vi "GoToWavelength.vi"(8 "error in (no error)":errorcluster, 10 "Wavelength":dbl, 11 "HRS_Spectrometer in":refnum<class "HRS_Spectrometer.lvclass">) -> (0 "error out":errorcluster, 3 "HRS_Spectrometer out":refnum<class "HRS_Spectrometer.lvclass">)   [LabVIEW 2023, in "HRS_Spectrometer.lvlib" / "HRS_Spectrometer.lvclass"]
uses:
  HRS_Spectrometer.lvclass
  HRS_Spectrometer.lvclass/HRS_Spectrometer.ctl
  <vilib>/Instr/_visa.llb/Select Event Type.ctl
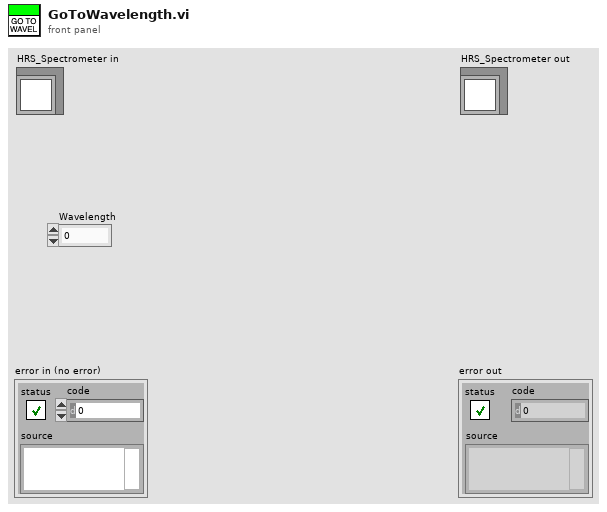
[diagram p1: front panel]
types:
  T1 = typedef "Select Event Type.ctl" = u32
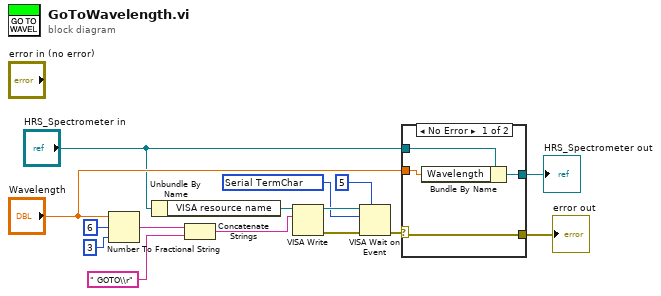
[diagram p0: block diagram]
diagram:
  w4 = T1 1073684516 items=["Service Request"=1073684491, "Trigger"=3221168138, "Clear"=1073684493, "VXI Signal"=1073684512, "VXI/VME Interrupt"=3221168161, "VXI/VME Sysfail"=1073684509, "VXI/VME Sysreset"=1073684510, "GPIB CIC"=1073684498, "GPIB Talk"=1073684499, "GPIB Listen"=1073684500, "PXI Interrupt"=1073684514, "Serial Break"=1073684515, "Serial TermChar"=1073684516, "Serial CTS"=1073684521, "Serial DSR"=1073684522, "Serial DCD"=1073684524, "Serial RI"=1073684526, "Serial Character"=1073684533, "USB Interrupt"=1073684535, "All Enabled"=1073709055] ("Event Type")
  n1 = Number To Fractional String(number="Wavelength", width (-)=i16 6, precision (6)=i16 3) -> (F-format string=w8:string)  [unwired: 1 in]
  n2 = Unbundle By Name("HRS_Spectrometer in") -> ("VISA resource name"=w10:refnum<visa-resource-name>)
  n3 = Concatenate Strings(w8, " GOTO\\r") -> (w7:string)
  n4 = VISA Write(VISA resource name=w10, write buffer=w7) -> (VISA resource name out=w6:refnum<visa-resource-name>, error out=w3:errorcluster)  [unwired: 1 in, 1 out]
  n5 = VISA Wait on Event(7:u32 5 ("timeout (0)"), 8:w3, 10:w4, 11:w6) -> (0:w2:errorcluster)  [unwired: 1 in, 3 out]
  n6 = case shown="No Error" w2 {
    selector: w2 -> [w16 w20]
    tunnel: "HRS_Spectrometer in" -> [w19 w21]
    tunnel: "Wavelength" -> [w18 _]
    tunnel: [w17 w21] -> w12
    tunnel: [w16 w20] -> w1
    frame No Error {
      n7 = Bundle By Name(cluster=w19, "Wavelength"=w18) -> (w17:refnum<class "HRS_Spectrometer.lvclass">)
    }
    frame Error {
    }
  }
  "error out" <- w1
  "HRS_Spectrometer out" <- w12
